vi "APS set point table 4DL.vi"(8 "error in (no error)":errorcluster caption="错误输入（无错误）", 9 "Point":T1, 10 "Index":i32, 11 "Axis_ID_Array":i32) -> (0 "error out":errorcluster caption="错误输出", 1 "Point out":T1, 2 "function return":i32, 3 "Axis_ID_Array out":i32)   [LabVIEW 2011, in "APS168.lvlib"]
doc: "I32 FNTYPE APS_set_point_table_4DL( I32 *Axis_ID_Array, I32 Index, PNT_DATA_4DL *Point );"
uses:
  APS168.lvlib
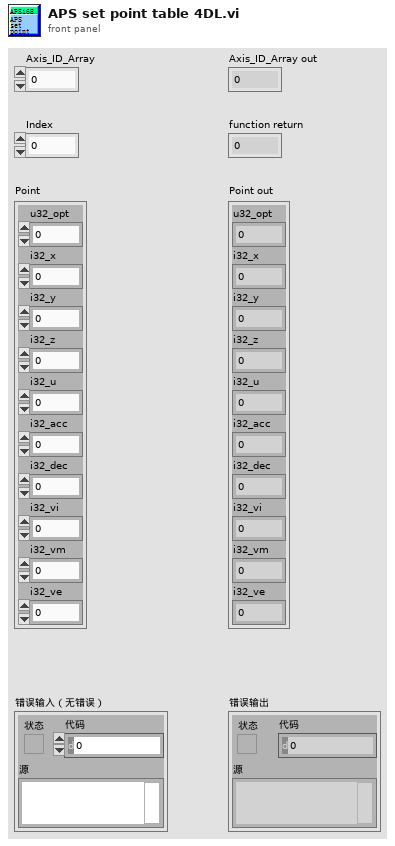
[diagram p1: front panel]
types:
  T1 = cluster{"u32_opt":u32, "i32_x":i32, "i32_y":i32, "i32_z":i32, "i32_u":i32, "i32_acc":i32, "i32_dec":i32, "i32_vi":i32, "i32_vm":i32, "i32_ve":i32}
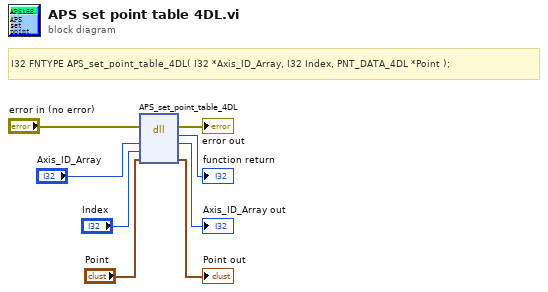
[diagram p0: block diagram]
diagram:
  # "I32 FNTYPE APS_set_point_table_4DL( I32 *Axis_ID_Array, I32 Index, PNT_DATA_4DL *Point );"
  n1 = dll-call lib="PTH1Labs E软件ADLINK 204CAPS_1_7_1_LIB line 连续运动204APS168.*" fn="APS_set_point_table_4DL"(error in="error in (no error)", "Axis_ID_Array"="Axis_ID_Array", "Index"="Index", "Point"="Point") -> (error out=→"error out":errorcluster, →"function return":i32, "Axis_ID_Array"=→"Axis_ID_Array out":i32, "Point"=→"Point out":T1)  [unwired: 3 in, 1 out]
